vi "MISC 3 Button Dialog.vi"(0 "Message":string, 5 "Button 1 Text (Run)":string="Run", 7 "Button 2 Text (Add)":string="Add", 9 "Button 3 Text (Cancel)":string="Cancel") -> (4 "Button Number":i32)   [LabVIEW 2011]
panel:
  in  "Button 2":bool
  in  "Button 3":bool
  in  "Goto":bool
  out "Error Out":errorcluster
  in  "Error In (no error)":errorcluster
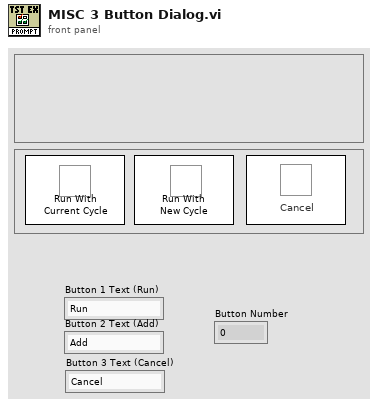
[diagram p1: front panel]
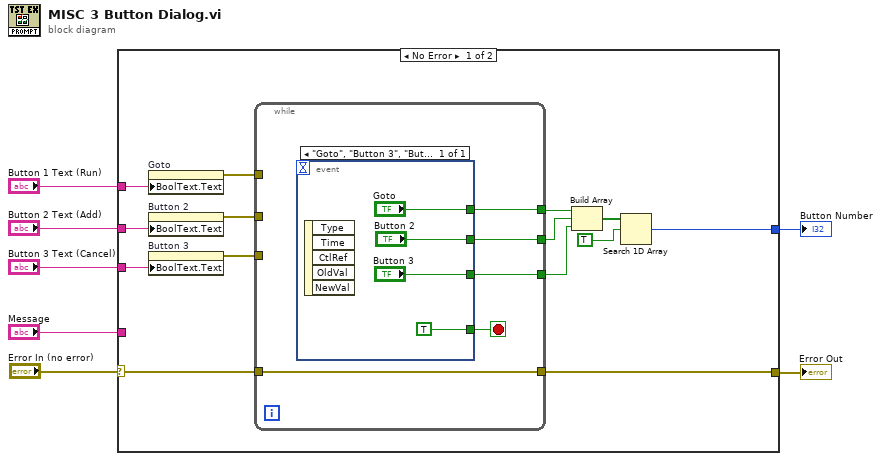
[diagram p0: block diagram]
diagram:
  n1 = case shown="No Error" "Error In (no error)" {
    selector: "Error In (no error)" -> [w20 w31]
    tunnel: [w21 w31] -> w7
    tunnel: "Button 1 Text (Run)" -> [w19 _]
    tunnel: "Button 2 Text (Add)" -> [w12 _]
    tunnel: "Message" -> [_ _]
    tunnel: "Button 3 Text (Cancel)" -> [w11 _]
    tunnel: [w13 _] -> w1
    frame No Error {
      n2 = property on="Goto" class="Bool"("BoolText.Text"=w19) -> (error out=w10:errorcluster)  [unwired: 2 in, 1 out]
      n3 = property on="Button 2" class="Bool"("BoolText.Text"=w12) -> (error out=w9:errorcluster)  [unwired: 2 in, 1 out]
      n4 = property on="Button 3" class="Bool"("BoolText.Text"=w11) -> (error out=w8:errorcluster)  [unwired: 2 in, 1 out]
      n5 = while {
        tunnel: [w24] -> w17
        tunnel: [w26] -> w21
        tunnel: w20 -> [w26]
        tunnel: [w23] -> w18
        tunnel: [w22] -> w16
        tunnel: w10 -> [_]
        tunnel: w9 -> [_]
        tunnel: w8 -> [_]
        stop <- w25 stop-if-true
        n6 = event shown="[0] \"Goto\", \"Button 3\", \"Button 2\": Value Change" {
          selector: _ -> [_]
          dyn-events: _ -> [_]
          timeout: _ -> [_]
          tunnel: [TRUE] -> w25
          tunnel: ["Button 2"] -> w24
          tunnel: ["Goto"] -> w23
          tunnel: ["Button 3"] -> w22
          event "Goto", "Button 3", "Button 2": Value Change {
            n7 = event-data() -> ()  [unwired: 6 out]
          }
        }
      }
      n8 = Build Array(w18, w17, w16) -> (w15:bool[])
      n9 = Search 1D Array(1D array=w15, element=TRUE) -> (index of element=w13:i32)  [unwired: 1 out]
    }
    frame Error {
    }
  }
  "Error Out" <- w7
  "Button Number" <- w1
